vi "Check Window Existence.vi"(8 "error in (no error)":errorcluster caption="错误输入（无错误）", 10 "Window Name":string, 11 "User Interface 输入":refnum<class "User Interface.lvclass">) -> (0 "error out":errorcluster caption="错误输出", 2 "已存在？":bool, 3 "User Interface 输出":refnum<class "User Interface.lvclass">)   [LabVIEW 2018, in "MainInterface.lvlib" / "User Interface.lvclass"]
uses:
  User Interface.lvclass
  User Interface.lvclass/User Interface.ctl
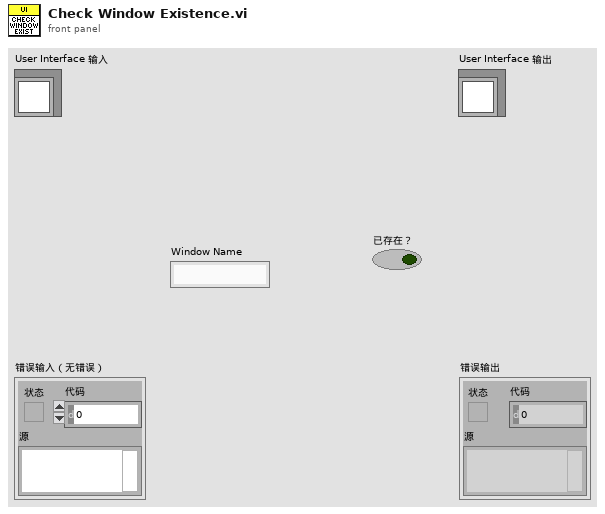
[diagram p1: front panel]
types:
  T1 = typedef "MainInterface.lvlib/Register Window Argument--cluster.ctl" = cluster{"Name":string, "Reference":refnum<vi>, "Message Queue":refnum<class "Delacor_lib_QMH_Message Queue.lvclass">}
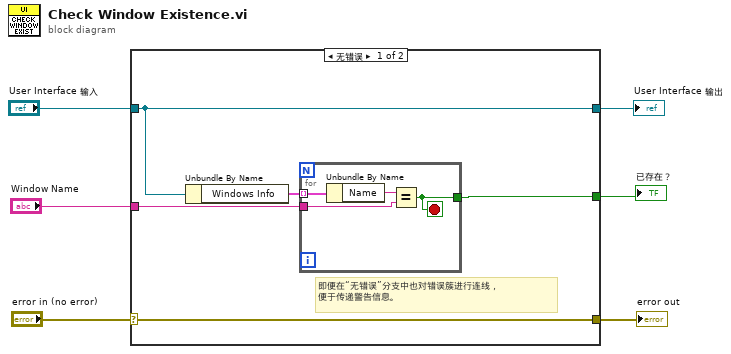
[diagram p0: block diagram]
diagram:
  n1 = case shown="无错误" "error in (no error)" {
    selector: "error in (no error)" -> [w11 w17]
    tunnel: [w11 w17] -> w5
    tunnel: [w10 w16] -> w3
    tunnel: "User Interface 输入" -> [w10 w16]
    tunnel: "Window Name" -> [w8 _]
    tunnel: [w7 _] -> w1
    frame No Error {
      # "即便在“无错误”分支中也对错误簇进行连线，\n便于传递警告信息。"
      n2 = Unbundle By Name(w10) -> ("Windows Info"=w9:T1[])
      n3 = for {
        tunnel: w9 -> [w15] mode=indexing
        tunnel: w8 -> [w13]
        tunnel: [w12] -> w7
        stop <- w12 stop-if-true
        n4 = Unbundle By Name(w15) -> ("Name"=w14:string)
        n5 = Equal?(x=w14, y=w13) -> (x = y?=w12:bool)
      }
    }
    frame Error {
    }
  }
  "error out" <- w5
  "User Interface 输出" <- w3
  "已存在？" <- w1
